vi "Atualiza_array_calibracao.vi"(8 "error in (no error)":errorcluster, 11 "refnum":T2) -> (0 "error out":errorcluster, 2 "Instrumentos":T1, 3 "refnum out":T2)   [LabVIEW 2019]
uses:
  <vilib>/Utility/config.llb/Config Data RefNum.ctl
  padrao_array_cluster_calibracao.ctl
  <vilib>/Utility/config.llb/Read Key (String).vi
  <vilib>/Utility/config.llb/Read Key (Double).vi
  <vilib>/Utility/config.llb/NI_LVConfig.lvlib
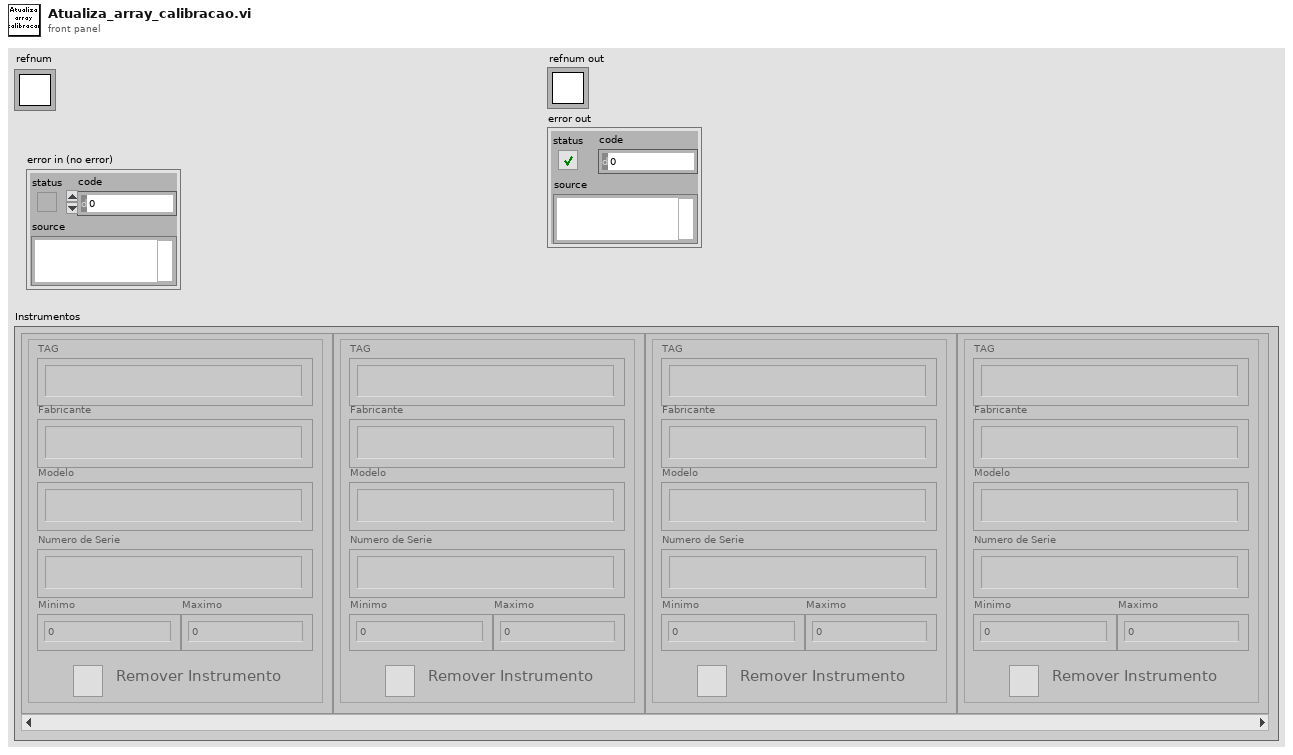
[diagram p1: front panel]
types:
  T1 = typedef "padrao_array_cluster_calibracao.ctl" = cluster{"TAG":string, "Minimo":dbl, "Fabricante":string, "Maximo":dbl, "remover_dipositvo":bool, "Modelo":string, "Numero de Serie":string}[]
  T2 = typedef "NI_LVConfig.lvlib/Config Data RefNum.ctl" = refnum<k1>
  T3 = cluster{"TAG":string, "Minimo":dbl, "Fabricante":string, "Maximo":dbl, "remover_dipositvo":bool, "Modelo":string, "Numero de Serie":string}
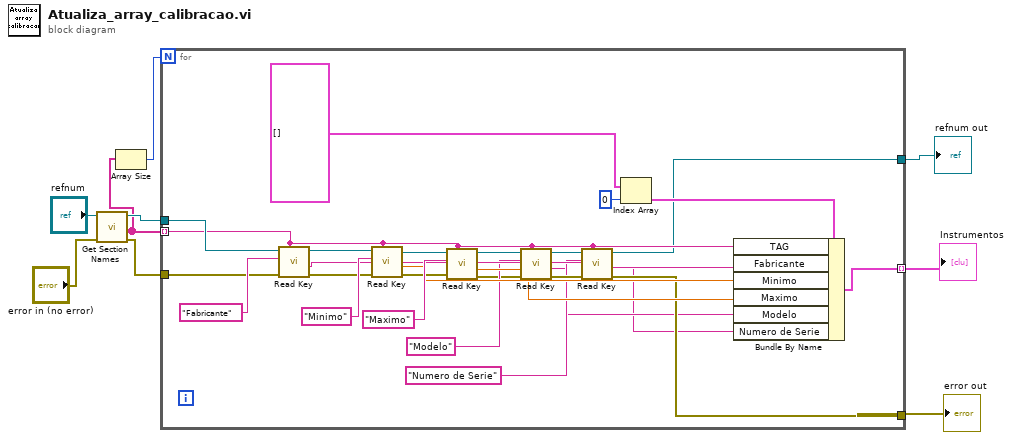
[diagram p0: block diagram]
diagram:
  n1 = call <vilib>:"Get Section Names.vi"("error in (no error)"="error in (no error)", "refnum"="refnum") -> ("error out"=w6:errorcluster, "section names"=w8:string[], "refnum out"=w9:T2)  [unwired: 7 in]
  n2 = Array Size(array=w8) -> (size(s)=w7:i32)
  n3 = for {
    N: w7 -> [_]
    tunnel: w8 -> [w20] mode=indexing
    tunnel: w9 -> [w36]
    tunnel: [w13] -> w3
    tunnel: [w14] -> w2
    tunnel: w6 -> [w26]
    tunnel: [w25] -> w1 mode=indexing
    n4 = call-poly <vilib>:"Read Key.vi"("section"=w20, "error in (no error)"=w26, "key"="Fabricante", "refnum"=w36) -> ("error out"=w28:errorcluster, "value"=w31:string, "refnum out"=w29:T2)  [unwired: 4 in, 1 out]
    n5 = call-poly <vilib>:"Read Key.vi"("section"=w20, "error in (no error)"=w28, "key"="Minimo", "refnum"=w29) -> ("error out"=w27:errorcluster, "value"=w30:dbl, "refnum out"=w32:T2)  [unwired: 4 in, 1 out]
    n6 = call-poly <vilib>:"Read Key.vi"("section"=w20, "error in (no error)"=w27, "key"="Maximo", "refnum"=w32) -> ("error out"=w16:errorcluster, "value"=w21:dbl, "refnum out"=w18:T2)  [unwired: 4 in, 1 out]
    n7 = call-poly <vilib>:"Read Key.vi"("section"=w20, "error in (no error)"=w16, "key"="Modelo", "refnum"=w18) -> ("error out"=w15:errorcluster, "value"=w11:string, "refnum out"=w17:T2)  [unwired: 4 in, 1 out]
    n8 = call-poly <vilib>:"Read Key.vi"("section"=w20, "error in (no error)"=w15, "key"="Numero de Serie", "refnum"=w17) -> ("error out"=w14:errorcluster, "value"=w10:string, "refnum out"=w13:T2)  [unwired: 4 in, 1 out]
    n9 = Index Array(array=T1 [] ("Instrumentos"), index=0) -> (element=w22:T3)
    n10 = Bundle By Name(cluster=w22, "TAG"=w20, "Fabricante"=w31, "Minimo"=w30, "Maximo"=w21, "Modelo"=w11, "Numero de Serie"=w10) -> (w25:T3)
  }
  "refnum out" <- w3
  "error out" <- w2
  "Instrumentos" <- w1
